vi "oct-scan_ctl.vi"() -> ()   [LabVIEW 2015]
panel:
  in  "y fall":dbl
  in  "y rise":dbl
  in  "y off":dbl(slide) scale=-1.0..1.0
  in  "y amp":dbl(slide) scale=-1.0..1.0
  in  "VISA resource name":refnum<visa-resource-name>="COM5"
  in  "f_scan kHz":dbl=2.691 format="%.3f"
  in  "f_ref kHz":dbl=425.0 format="%.3f"
  in  "x amplitude":dbl(slide)=0.1 scale=0.0..1.5
  in  "phase":dbl(slide) scale=-3.0..3.0
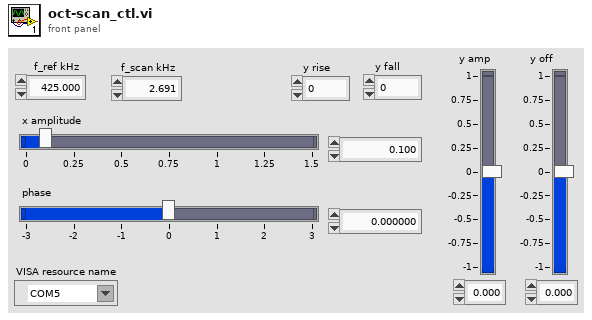
[diagram p1: front panel]
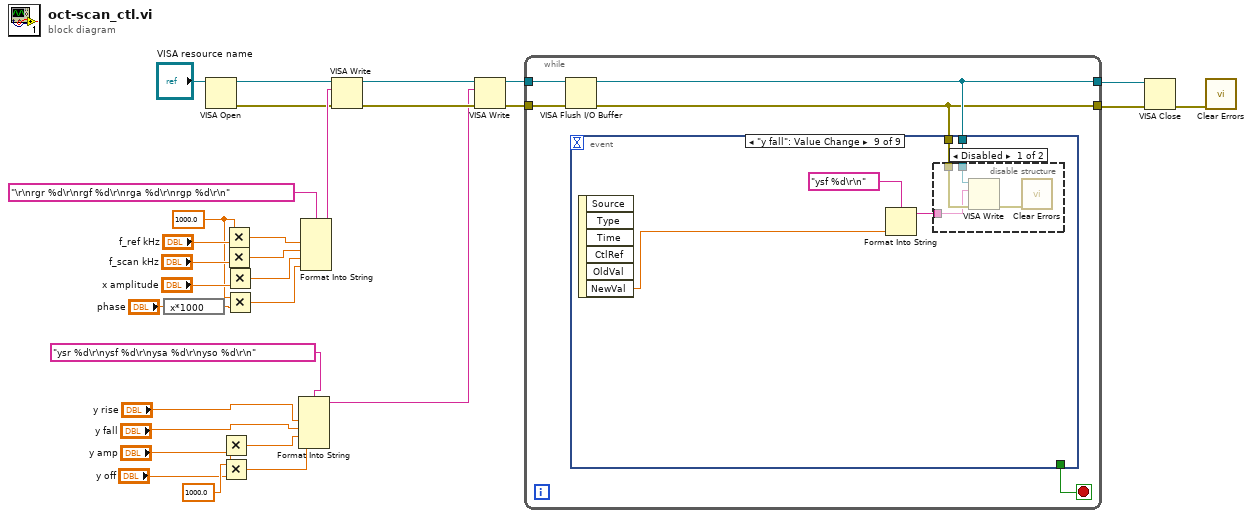
[diagram p0: block diagram]
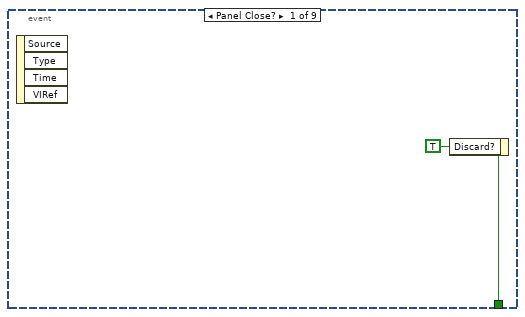
[diagram p2: hidden frame]
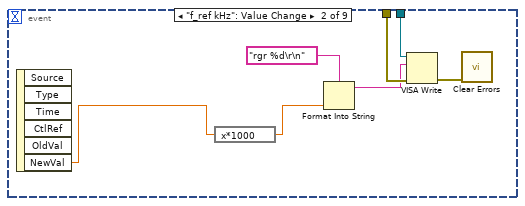
[diagram p3: hidden frame]
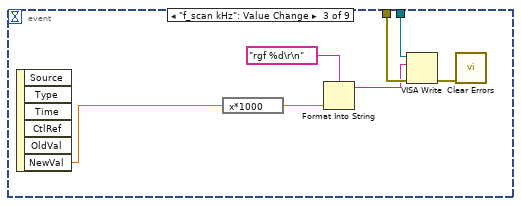
[diagram p4: hidden frame]
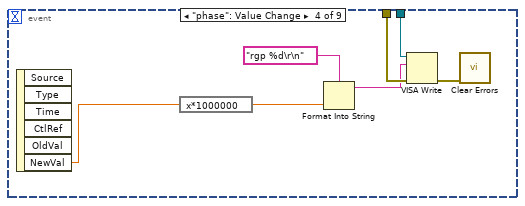
[diagram p5: hidden frame]
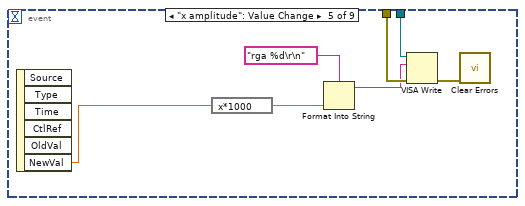
[diagram p6: hidden frame]
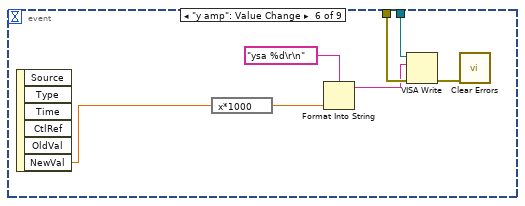
[diagram p7: hidden frame]
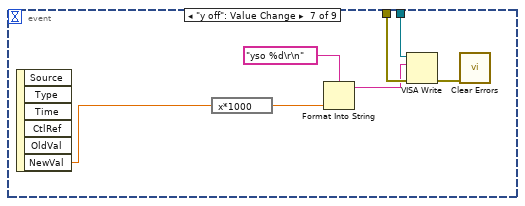
[diagram p8: hidden frame]
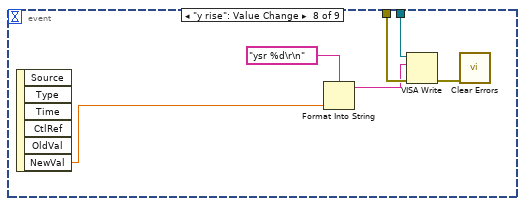
[diagram p9: hidden frame]
diagram:
  w8 = 1000.0
  w14 = 1000.0
  n1 = expression code="x*1000"("phase") -> (w15:dbl)
  n2 = VISA Open(VISA resource name="VISA resource name") -> (VISA resource name=w22:refnum<visa-resource-name>, error out=w21:errorcluster)  [unwired: 4 in]
  n3 = Multiply(x=w8, y="y amp") -> (x*y=w4:dbl)
  n4 = Multiply(x=w8, y="y off") -> (x*y=w3:dbl)
  n5 = Multiply(x=w14, y="f_ref kHz") -> (x*y=w20:dbl)
  n6 = Multiply(x=w14, y="f_scan kHz") -> (x*y=w19:dbl)
  n7 = Multiply(x=w14, y="x amplitude") -> (x*y=w18:dbl)
  n8 = Multiply(x=w14, y=w15) -> (x*y=w17:dbl)
  n9 = Format Into String(format string="ysr %d\r\nysf %d\r\nysa %d\r\nyso %d\r\n", "y rise", "y fall", w4, w3) -> (resulting string=w9:string)  [unwired: 2 in, 1 out]
  n10 = Format Into String(format string="\r\nrgr %d\r\nrgf %d\r\nrga %d\r\nrgp %d\r\n", w20, w19, w18, w17) -> (resulting string=w23:string)  [unwired: 2 in, 1 out]
  n11 = VISA Write(VISA resource name=w22, write buffer=w23, error in (no error)=w21) -> (VISA resource name out=w12:refnum<visa-resource-name>, error out=w13:errorcluster)  [unwired: 1 out]
  n12 = VISA Write(VISA resource name=w12, write buffer=w9, error in (no error)=w13) -> (VISA resource name out=w11:refnum<visa-resource-name>, error out=w10:errorcluster)  [unwired: 1 out]
  n13 = while {
    tunnel: w11 -> [w35]
    tunnel: [w34] -> w30
    tunnel: w10 -> [w33]
    tunnel: [w32] -> w29
    stop <- w36 stop-if-true
    n14 = VISA Flush I/O Buffer(VISA resource name=w35, error in (no error)=w33) -> (VISA resource name out=w34:refnum<visa-resource-name>, error out=w32:errorcluster)  [unwired: 1 in]
    n15 = event shown="[8] \"y fall\": Value Change" {
      selector: _ -> [_ _ _ _ _ _ _ _ _]
      dyn-events: _ -> [_ _ _ _ _ _ _ _ _]
      timeout: _ -> [_ _ _ _ _ _ _ _ _]
      tunnel: [w37 _ _ _ _ _ _ _ _] -> w36
      tunnel: w34 -> [_ w44 w51 w58 w65 w72 w79 w85 w90]
      tunnel: w32 -> [_ w43 w50 w57 w64 w71 w78 w84 w89]
      event Panel Close? {
        w37 = TRUE ("Discard?")
        n16 = event-data() -> ()  [unwired: 1 in, 4 out]
        n17 = event-data("Discard?"=w37) -> ()  [unwired: 1 in, 1 out]
      }
      event "f_ref kHz": Value Change {
        n18 = event-data() -> ("NewVal"=w39:dbl)  [unwired: 1 in, 5 out]
        n19 = expression code="x*1000"(w39) -> (w38:dbl)
        n20 = Format Into String(format string="rgr %d\r\n", w38) -> (resulting string=w41:string)  [unwired: 2 in, 1 out]
        n21 = VISA Write(VISA resource name=w44, write buffer=w41, error in (no error)=w43) -> (error out=w40:errorcluster)  [unwired: 2 out]
        n22 = call <vilib>:"Clear Errors.vi"("error in (no error)"=w40) -> ()  [unwired: 5 in, 2 out]
      }
      event "f_scan kHz": Value Change {
        n23 = event-data() -> ("NewVal"=w48:dbl)  [unwired: 1 in, 5 out]
        n24 = expression code="x*1000"(w48) -> (w46:dbl)
        n25 = Format Into String(format string="rgf %d\r\n", w46) -> (resulting string=w45:string)  [unwired: 2 in, 1 out]
        n26 = VISA Write(VISA resource name=w51, write buffer=w45, error in (no error)=w50) -> (error out=w47:errorcluster)  [unwired: 2 out]
        n27 = call <vilib>:"Clear Errors.vi"("error in (no error)"=w47) -> ()  [unwired: 5 in, 2 out]
      }
      event "phase": Value Change {
        n28 = event-data() -> ("NewVal"=w52:dbl)  [unwired: 1 in, 5 out]
        n29 = expression code="x*1000000"(w52) -> (w53:dbl)
        n30 = Format Into String(format string="rgp %d\r\n", w53) -> (resulting string=w55:string)  [unwired: 2 in, 1 out]
        n31 = VISA Write(VISA resource name=w58, write buffer=w55, error in (no error)=w57) -> (error out=w54:errorcluster)  [unwired: 2 out]
        n32 = call <vilib>:"Clear Errors.vi"("error in (no error)"=w54) -> ()  [unwired: 5 in, 2 out]
      }
      event "x amplitude": Value Change {
        n33 = event-data() -> ("NewVal"=w62:dbl)  [unwired: 1 in, 5 out]
        n34 = expression code="x*1000"(w62) -> (w59:dbl)
        n35 = Format Into String(format string="rga %d\r\n", w59) -> (resulting string=w61:string)  [unwired: 2 in, 1 out]
        n36 = VISA Write(VISA resource name=w65, write buffer=w61, error in (no error)=w64) -> (error out=w60:errorcluster)  [unwired: 2 out]
        n37 = call <vilib>:"Clear Errors.vi"("error in (no error)"=w60) -> ()  [unwired: 5 in, 2 out]
      }
      event "y amp": Value Change {
        n38 = event-data() -> ("NewVal"=w69:dbl)  [unwired: 1 in, 5 out]
        n39 = expression code="x*1000"(w69) -> (w67:dbl)
        n40 = Format Into String(format string="ysa %d\r\n", w67) -> (resulting string=w68:string)  [unwired: 2 in, 1 out]
        n41 = VISA Write(VISA resource name=w72, write buffer=w68, error in (no error)=w71) -> (error out=w66:errorcluster)  [unwired: 2 out]
        n42 = call <vilib>:"Clear Errors.vi"("error in (no error)"=w66) -> ()  [unwired: 5 in, 2 out]
      }
      event "y off": Value Change {
        n43 = event-data() -> ("NewVal"=w76:dbl)  [unwired: 1 in, 5 out]
        n44 = expression code="x*1000"(w76) -> (w74:dbl)
        n45 = Format Into String(format string="yso %d\r\n", w74) -> (resulting string=w75:string)  [unwired: 2 in, 1 out]
        n46 = VISA Write(VISA resource name=w79, write buffer=w75, error in (no error)=w78) -> (error out=w73:errorcluster)  [unwired: 2 out]
        n47 = call <vilib>:"Clear Errors.vi"("error in (no error)"=w73) -> ()  [unwired: 5 in, 2 out]
      }
      event "y rise": Value Change {
        n48 = event-data() -> ("NewVal"=w80:dbl)  [unwired: 1 in, 5 out]
        n49 = Format Into String(format string="ysr %d\r\n", w80) -> (resulting string=w82:string)  [unwired: 2 in, 1 out]
        n50 = VISA Write(VISA resource name=w85, write buffer=w82, error in (no error)=w84) -> (error out=w81:errorcluster)  [unwired: 2 out]
        n51 = call <vilib>:"Clear Errors.vi"("error in (no error)"=w81) -> ()  [unwired: 5 in, 2 out]
      }
      event "y fall": Value Change {
        n52 = event-data() -> ("NewVal"=w86:dbl)  [unwired: 1 in, 5 out]
        n53 = Format Into String(format string="ysf %d\r\n", w86) -> (resulting string=w87:string)  [unwired: 2 in, 1 out]
        n54 = disable-structure shown="Disabled" {
          disable-tunnel: w90 -> [w94 _]
          disable-tunnel: w89 -> [w93 _]
          disable-tunnel: w87 -> [w92 _]
          frame Disabled {
            n55 = VISA Write(VISA resource name=w94, write buffer=w92, error in (no error)=w93) -> (error out=w91:errorcluster)  [unwired: 2 out]
            n56 = call <vilib>:"Clear Errors.vi"("error in (no error)"=w91) -> ()  [unwired: 5 in, 2 out]
          }
          frame Enabled {
          }
        }
      }
    }
  }
  n57 = VISA Close(VISA resource name=w30, error in (no error)=w29) -> (error out=w28:errorcluster)
  n58 = call <vilib>:"Clear Errors.vi"("error in (no error)"=w28) -> ()  [unwired: 5 in, 2 out]
